vi "PWM_test.vi"(0 "Input buffer size":u32=16384, 3 "Stop Button":bool, 5 "Select COM port":refnum<visa-resource-name>="COM3", 9 "baud rate":u32=1200000, 11 "Period 2":u16=10 min=10 max=65000 step=1, 12 "% Duty Cycle":dbl=5.0 min=0.01 max=99.99 step=0.01, 14 "1. Apply Command":bool) -> (1 "Apply Ind":bool, 4 "RESET USB":bool, 6 "Connected to:":string, 8 "Frequency Hz":dbl, 10 "Message":string, 15 "Waveform Graph":dynamicdata(graph))   [LabVIEW 2012]
panel:
  out "Duty cycle":string
  out "Period":string
  out "T command Bytes sent":dbl
  out "Number of bytes written":dbl
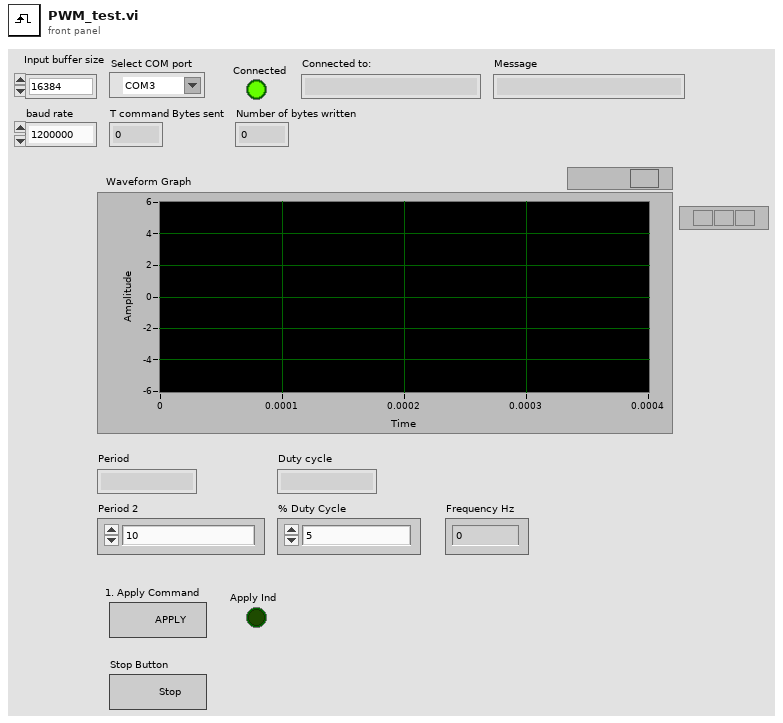
[diagram p1: front panel]
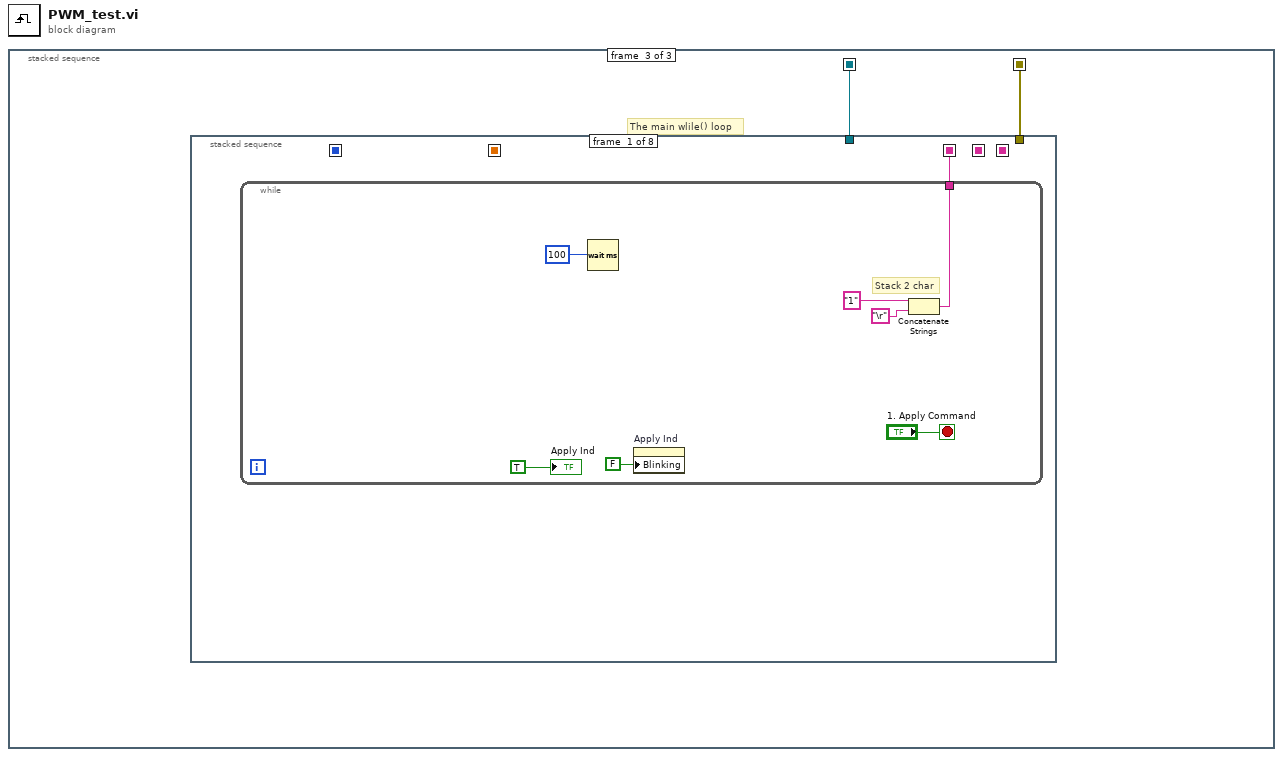
[diagram p0: block diagram]
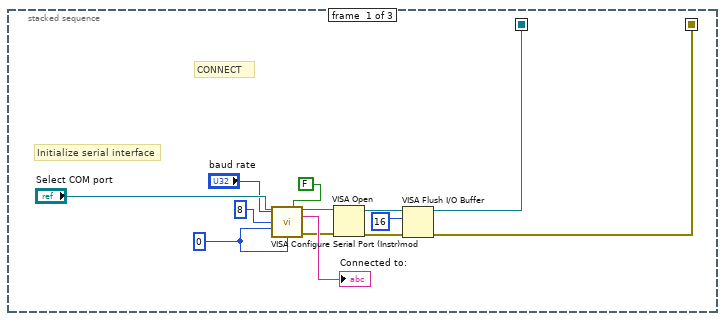
[diagram p2: hidden frame]
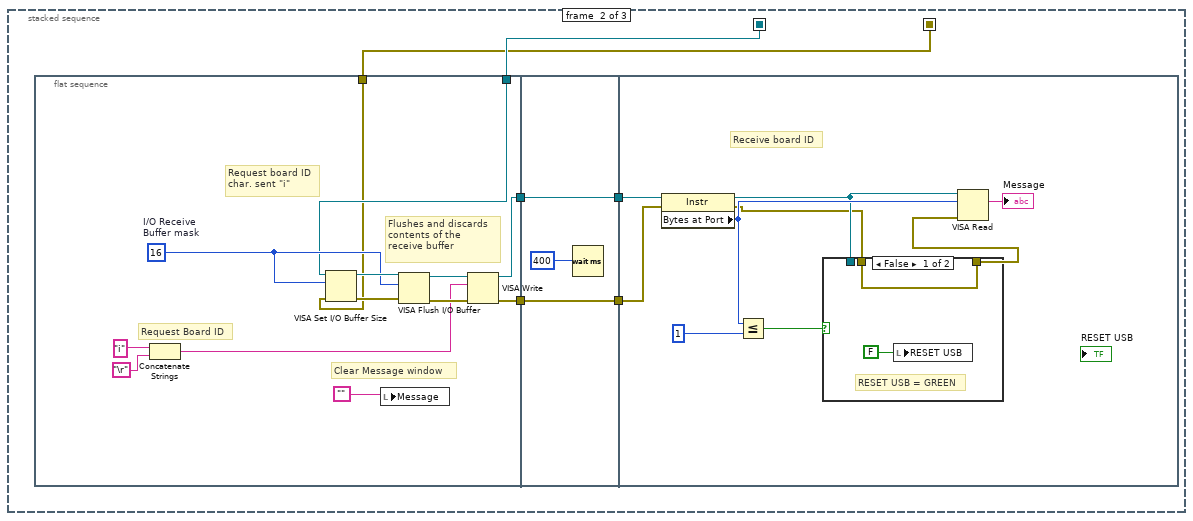
[diagram p3: hidden frame]
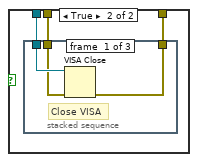
[diagram p4: hidden frame]
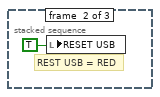
[diagram p5: hidden frame]
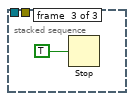
[diagram p6: hidden frame]
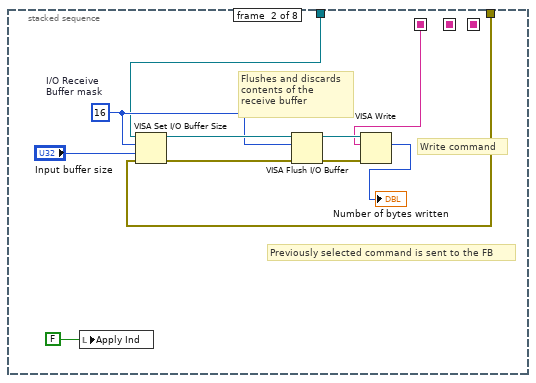
[diagram p7: hidden frame]
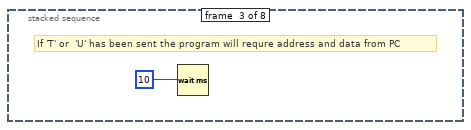
[diagram p8: hidden frame]
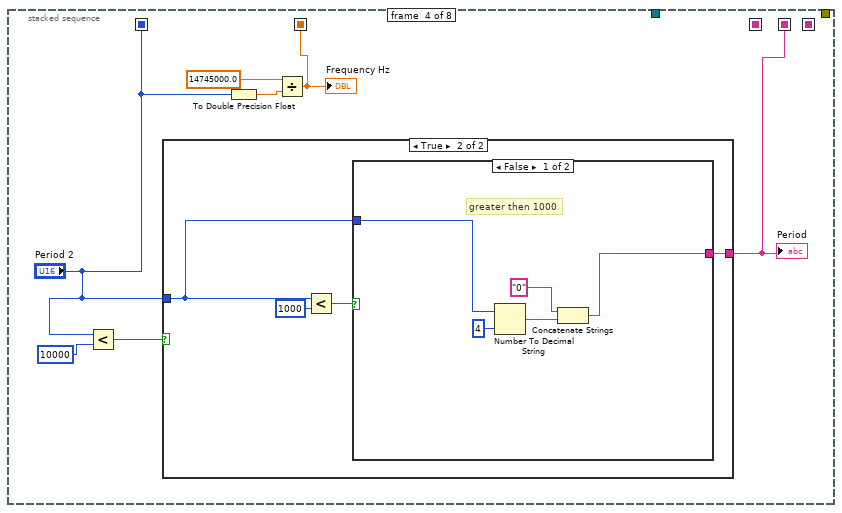
[diagram p9: hidden frame]
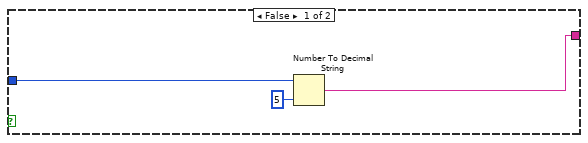
[diagram p10: hidden frame]
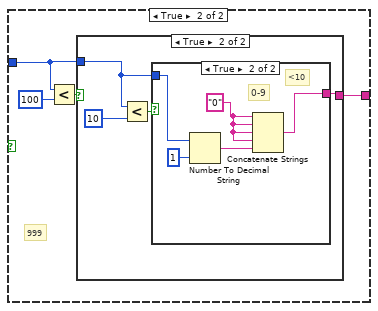
[diagram p11: hidden frame]
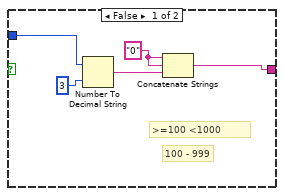
[diagram p12: hidden frame]
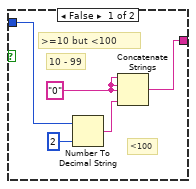
[diagram p13: hidden frame]
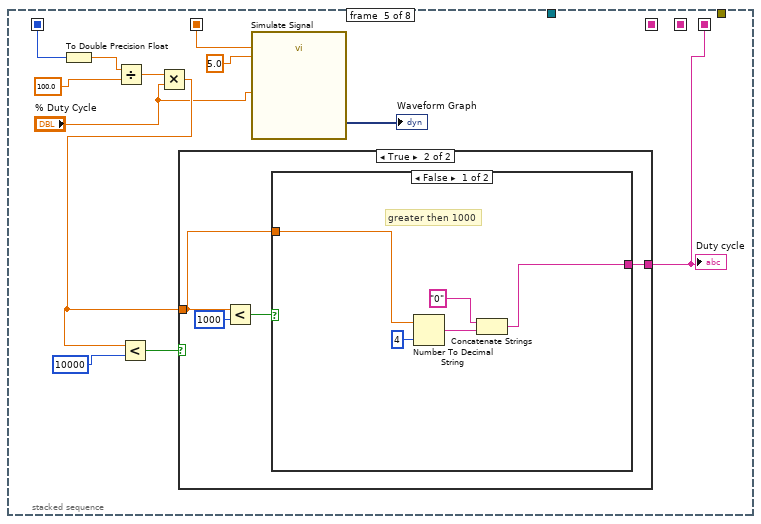
[diagram p14: hidden frame]
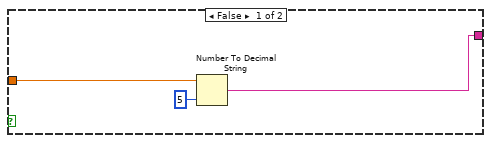
[diagram p15: hidden frame]
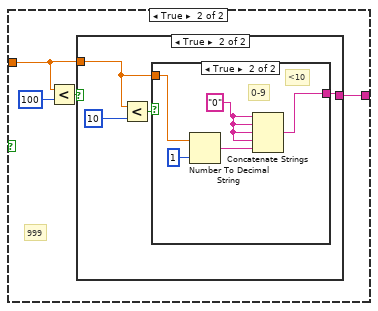
[diagram p16: hidden frame]
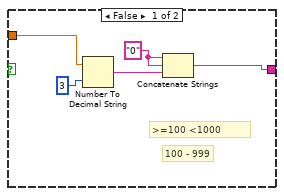
[diagram p17: hidden frame]
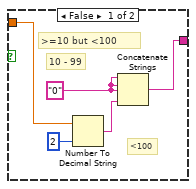
[diagram p18: hidden frame]
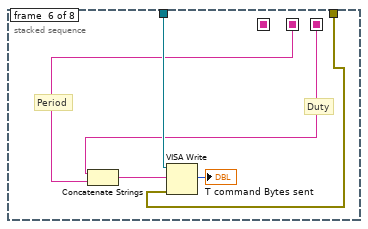
[diagram p19: hidden frame]
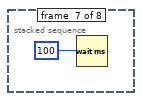
[diagram p20: hidden frame]
diagram:
  n1 = stacked-sequence {
    seq-local: [w2 _ _] -> [_ w19 w55]
    seq-local: [w1 _ _] -> [_ w18 w56]
    frame #0 {
      w4 = 0
      # "CONNECT"
      # "Initialize serial interface"
      n2 = call "VISA Configure Serial Port (Instr)mod.vi"("VISA resource name"="Select COM port", "Enable Termination\nChar (T)"=FALSE, "baud rate (9600)"="baud rate", "data bits (8)"=8, "parity (0:none)"=w4, "flow control (0:none)"=w4) -> ("VISA resource name out"=w8:refnum<visa-resource-name>, "Name"=→"Connected to:":string, "error out"=w7:errorcluster)  [unwired: 6 in, 1 out]
      n3 = VISA Open(error in (no error)=w7, VISA resource name=w8) -> (VISA resource name=w6:refnum<visa-resource-name>, error out=w5:errorcluster)  [unwired: 3 out]
      n4 = VISA Flush I/O Buffer(VISA resource name=w6, mask (16)=u16 16 ("Maskieren (16)"), error in (no error)=w5) -> (VISA resource name out=w2:refnum<visa-resource-name>, error out=w1:errorcluster)
    }
    frame #1 {
      n5 = flat-sequence {
        tunnel: w19 -> [w26]
        tunnel: w18 -> [w25]
        tunnel: [w24] -> w16
        tunnel: [w23] -> w14
        tunnel: [w34] -> w17
        tunnel: w16 -> [w34]
        tunnel: [w33] -> w15
        tunnel: w14 -> [w33]
        tunnel: w17 -> [w37]
        tunnel: w15 -> [w36]
        frame #0 {
          w28 = u16 16  # I/O Receive Buffer mask
          # "Clear Message window"
          # "Request board ID\nchar. sent \"i\""
          # "Request Board ID"
          # "Flushes and discards \ncontents of the \nreceive buffer"
          n6 = Concatenate Strings("i", "\r") -> (w27:string)
          n7 = VISA Set I/O Buffer Size(VISA resource name=w26, mask (16)=w28, error in (no error)=w25) -> (VISA resource name out=w30:refnum<visa-resource-name>, error out=w29:errorcluster)  [unwired: 1 in]
          n8 = local write "Message"("") -> ()
          n9 = VISA Flush I/O Buffer(VISA resource name=w30, mask (16)=w28, error in (no error)=w29) -> (VISA resource name out=w32:refnum<visa-resource-name>, error out=w31:errorcluster)
          n10 = VISA Write(VISA resource name=w32, write buffer=w27, error in (no error)=w31) -> (VISA resource name out=w24:refnum<visa-resource-name>, error out=w23:errorcluster)  [unwired: 1 out]
        }
        frame #1 {
          n11 = Wait (ms)(milliseconds to wait=400) -> ()  [unwired: 1 out]
        }
        frame #2 {
          # "Receive board ID"
          n12 = property class="Instr"(reference=w37, error in=w36) -> (reference out=w41:refnum<visa-resource-name>, error out=w39:errorcluster, "Bytes at Port"=w43:u32)
          n13 = Less Or Equal?(x=w43, y=1) -> (x <= y?=w44:bool)
          n14 = case shown="False" w44 {
            tunnel: w41 -> [_ w49]
            tunnel: w39 -> [w45 w48]
            tunnel: [w45 w47] -> w38
            frame False {
              # "RESET USB = GREEN"
              n15 = local write "RESET USB"(FALSE) -> ()
            }
            frame True {
              n16 = stacked-sequence {
                tunnel: w49 -> [w52 _ _]
                tunnel: w48 -> [w51 _ _]
                tunnel: [w50 _ _] -> w47
                frame #0 {
                  # "Close VISA"
                  n17 = VISA Close(VISA resource name=w52, error in (no error)=w51) -> (error out=w50:errorcluster)
                }
                frame #1 {
                  # "REST USB = RED"
                  n18 = local write "RESET USB"(TRUE) -> ()
                }
                frame #2 {
                  n19 = Stop(stop? (T)=TRUE ("Stop? (T)")) -> ()
                }
              }
            }
          }
          n20 = VISA Read(VISA resource name=w41, byte count=w43, error in (no error)=w38) -> (read buffer=→"Message":string)  [unwired: 3 out]
        }
      }
    }
    frame #2 {
      # "The main wlile() loop"
      n21 = stacked-sequence {
        seq-local: [w57 _ _ _ _ _ _ _] -> [_ w68 _ _ _ _ _ _]
        seq-local: [_ _ _ w81 _ _ _ _] -> [_ _ _ _ _ w166 _ _]
        seq-local: [_ _ _ _ w128 _ _ _] -> [_ _ _ _ _ w167 _ _]
        seq-local: [_ _ _ "Period 2" _ _ _ _] -> [_ _ _ _ w127 _ _ _]
        seq-local: [_ _ _ w77 _ _ _ _] -> [_ _ _ _ w122 _ _ _]
        tunnel: w55 -> [_ w70 _ _ _ w171 _ w174]
        tunnel: w56 -> [_ w69 _ _ _ w170 _ _]
        frame #0 {
          n22 = while {
            tunnel: [w59] -> w57
            stop <- "1. Apply Command" stop-if-true
            # "Stack 2 char"
            n23 = Wait (ms)(milliseconds to wait=100) -> ()  [unwired: 1 out]
            n24 = property on="Apply Ind" class="Bool (strict)"("Blinking"=FALSE) -> ()  [unwired: 2 in, 2 out]
            n25 = Concatenate Strings("1", "\r") -> (w59:string)
            "Apply Ind" <- TRUE
          }
        }
        frame #1 {
          w71 = u16 16  # I/O Receive Buffer mask
          # "Write command"
          # "Previously selected command is sent to the FB"
          # "Flushes and discards \ncontents of the \nreceive buffer"
          n26 = local write "Apply Ind"(FALSE) -> ()
          n27 = VISA Set I/O Buffer Size(VISA resource name=w70, mask (16)=w71, size (4096)="Input buffer size", error in (no error)=w69) -> (VISA resource name out=w73:refnum<visa-resource-name>, error out=w72:errorcluster)
          n28 = VISA Flush I/O Buffer(VISA resource name=w73, mask (16)=w71, error in (no error)=w72) -> (VISA resource name out=w75:refnum<visa-resource-name>, error out=w74:errorcluster)
          n29 = VISA Write(VISA resource name=w75, write buffer=w68, error in (no error)=w74) -> (return count=→"Number of bytes written":u32)  [unwired: 2 out]
        }
        frame #2 {
          # "If 'T' or  'U' has been sent the program will requre address and data from PC"
          n30 = Wait (ms)(milliseconds to wait=10) -> ()  [unwired: 1 out]
        }
        frame #3 {
          n31 = Less?(x="Period 2", y=10000) -> (x < y?=w82:bool)
          n32 = case shown="True" w82 {
            tunnel: [w84 w90] -> w81
            tunnel: "Period 2" -> [w85 w87]
            frame False {
              n33 = Number To Decimal String(number=w85, width (-)=5) -> (decimal integer string=w84:string)
            }
            frame True {
              n34 = Less?(x=w87, y=1000) -> (x < y?=w88:bool)
              n35 = case shown="False" w88 {
                tunnel: [w91 w97] -> w90
                tunnel: w87 -> [w93 w96]
                frame False {
                  # "greater then 1000"
                  n36 = Number To Decimal String(number=w93, width (-)=4) -> (decimal integer string=w94:string)
                  n37 = Concatenate Strings("0", w94) -> (w91:string)
                }
                frame True {
                  # "999"
                  n38 = Less?(x=w96, y=100) -> (x < y?=w99:bool)
                  n39 = case shown="True" w99 {
                    tunnel: [w100 w105] -> w97
                    tunnel: w96 -> [w103 w106]
                    frame False {
                      w101 = "0"
                      # "100 - 999"
                      # ">=100 <1000"
                      n40 = Number To Decimal String(number=w103, width (-)=3) -> (decimal integer string=w102:string)
                      n41 = Concatenate Strings(w101, w101, w102) -> (w100:string)
                    }
                    frame True {
                      n42 = Less?(x=w106, y=10) -> (x < y?=w108:bool)
                      n43 = case shown="True" w108 {
                        tunnel: w106 -> [w111 w115]
                        tunnel: [w109 w116] -> w105
                        frame False {
                          w110 = "0"
                          # "10 - 99"
                          # ">=10 but <100"
                          # "<100"
                          n44 = Number To Decimal String(number=w111, width (-)=2) -> (decimal integer string=w112:string)
                          n45 = Concatenate Strings(w110, w110, w110, w112) -> (w109:string)
                        }
                        frame True {
                          w114 = "0"
                          # "0-9"
                          # "<10"
                          n46 = Number To Decimal String(number=w115, width (-)=1) -> (decimal integer string=w117:string)
                          n47 = Concatenate Strings(w114, w114, w114, w114, w117) -> (w116:string)
                        }
                      }
                    }
                  }
                }
              }
            }
          }
          "Period" <- w81
          n48 = To Double Precision Float(number="Period 2") -> (double precision float=w78:dbl)
          n49 = Divide(x=14745000.0, y=w78) -> (x/y=w77:dbl)
          "Frequency Hz" <- w77
        }
        frame #4 {
          n50 = To Double Precision Float(number=w127) -> (double precision float=w125:dbl)
          n51 = Divide(x=w125, y=100.0) -> (x/y=w124:dbl)
          n52 = Multiply(x=w124, y="% Duty Cycle") -> (x*y=w123:dbl)
          n53 = Less?(x=w123, y=10000) -> (x < y?=w129:bool)
          n54 = case shown="True" w129 {
            tunnel: [w131 w137] -> w128
            tunnel: w123 -> [w132 w134]
            frame False {
              n55 = Number To Decimal String(number=w132, width (-)=5) -> (decimal integer string=w131:string)
            }
            frame True {
              n56 = Less?(x=w134, y=1000) -> (x < y?=w135:bool)
              n57 = case shown="False" w135 {
                tunnel: [w138 w144] -> w137
                tunnel: w134 -> [w140 w143]
                frame False {
                  # "greater then 1000"
                  n58 = Number To Decimal String(number=w140, width (-)=4) -> (decimal integer string=w141:string)
                  n59 = Concatenate Strings("0", w141) -> (w138:string)
                }
                frame True {
                  # "999"
                  n60 = Less?(x=w143, y=100) -> (x < y?=w146:bool)
                  n61 = case shown="True" w146 {
                    tunnel: [w147 w152] -> w144
                    tunnel: w143 -> [w150 w153]
                    frame False {
                      w148 = "0"
                      # "100 - 999"
                      # ">=100 <1000"
                      n62 = Number To Decimal String(number=w150, width (-)=3) -> (decimal integer string=w149:string)
                      n63 = Concatenate Strings(w148, w148, w149) -> (w147:string)
                    }
                    frame True {
                      n64 = Less?(x=w153, y=10) -> (x < y?=w155:bool)
                      n65 = case shown="True" w155 {
                        tunnel: w153 -> [w158 w162]
                        tunnel: [w156 w163] -> w152
                        frame False {
                          w157 = "0"
                          # "10 - 99"
                          # ">=10 but <100"
                          # "<100"
                          n66 = Number To Decimal String(number=w158, width (-)=2) -> (decimal integer string=w159:string)
                          n67 = Concatenate Strings(w157, w157, w157, w159) -> (w156:string)
                        }
                        frame True {
                          w161 = "0"
                          # "0-9"
                          # "<10"
                          n68 = Number To Decimal String(number=w162, width (-)=1) -> (decimal integer string=w164:string)
                          n69 = Concatenate Strings(w161, w161, w161, w161, w164) -> (w163:string)
                        }
                      }
                    }
                  }
                }
              }
            }
          }
          "Duty cycle" <- w128
          n70 = call "Simulate Signal"("Duty Cycle (%)"="% Duty Cycle", "Frequency"=w122, "Amplitude"=5.0) -> ("Square"=→"Waveform Graph":dynamicdata)  [unwired: 11 in, 1 out]
        }
        frame #5 {
          # "Period"
          # "Duty"
          n71 = Concatenate Strings(w167, w166) -> (w168:string)
          n72 = VISA Write(VISA resource name=w171, write buffer=w168, error in (no error)=w170) -> (return count=→"T command Bytes sent":u32)  [unwired: 2 out]
        }
        frame #6 {
          n73 = Wait (ms)(milliseconds to wait=100) -> ()  [unwired: 1 out]
        }
        frame #7 {
          n74 = case shown="False" "Stop Button" {
            tunnel: w174 -> [_ w175]
            frame False {
            }
            frame True {
              n75 = stacked-sequence {
                tunnel: w175 -> [w177 _ w179 _]
                frame #0 {
                  n76 = call "g_send.vi"("Input buffer size"=16384, "USB Interface Name"=w177) -> ()  [unwired: 9 in, 1 out]
                }
                frame #1 {
                  n77 = Wait (ms)(milliseconds to wait=5) -> ()  [unwired: 1 out]
                }
                frame #2 {
                  n78 = VISA Close(VISA resource name=w179) -> ()  [unwired: 1 in, 1 out]
                }
                frame #3 {
                  n79 = Stop(stop? (T)=TRUE ("Stop? (T)")) -> ()
                }
              }
            }
          }
        }
      }
    }
  }
